vi "SCLN_IndexServer.vi"(1 "Server Name":string) -> (0 "Index":i32)   [LabVIEW 2015]
doc: "Find the index corresponding to\na server in the table of\nserver names. If the name doesn't exist, returns -1."
uses:
  SCLN_RW_Select.ctl
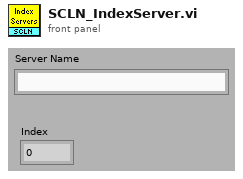
[diagram p1: front panel]
types:
  T1 = typedef "SCLN_RW_Select.ctl" = enum16{"Read", "Write"}
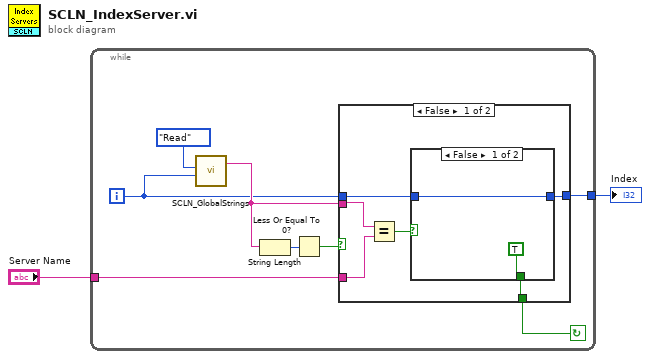
[diagram p0: block diagram]
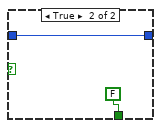
[diagram p2: hidden frame]
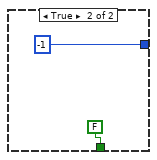
[diagram p3: hidden frame]
diagram:
  n1 = while {
    tunnel: [w7] -> w2
    tunnel: "Server Name" -> [w5]
    i -> [w3]
    stop <- w6 continue-if-true
    n2 = call "SCLN_GlobalStrings.vi"("Element"=w3, "Operation"=SCLN_RW_Select."Read" ("GBL_RW")) -> ("Read Value"=w4:string)  [unwired: 2 in, 1 out]
    n3 = String Length(string=w4) -> (length=w9:i32)
    n4 = Less Or Equal To 0?(x=w9) -> (x <= 0?=w8:bool)
    n5 = case shown="False" w8 {
      tunnel: [w12 -1] -> w7
      tunnel: [w11 FALSE] -> w6
      tunnel: w5 -> [w15 _]
      tunnel: w4 -> [w16 _]
      tunnel: w3 -> [w13 _]
      frame False {
        n6 = Equal?(x=w16, y=w15) -> (x = y?=w14:bool)
        n7 = case shown="False" w14 {
          tunnel: w13 -> [w17 w20]
          tunnel: [w17 w20] -> w12
          tunnel: [TRUE FALSE] -> w11
          frame False {
          }
          frame True {
          }
        }
      }
      frame True {
      }
    }
  }
  "Index" <- w2
